vi "Eval X-Y(t).vi"(4 "Formulas":string[](array[string])=["", ""], 5 "end":dbl=1.0 format="%.2f", 6 "start":dbl format="%.2f", 7 "number of points":u32=10) -> (0 "error":i32, 1 "ticks":u32, 2 "Y":dbl[](array[numeric]) format="%.2f", 3 "X":dbl[](array[numeric]) format="%.2f")   [LabVIEW 2020, in "NI_Gmath.lvlib"]
doc: "Calculates the values of a function (f(t), g(t)), where t runs over an interval. Both components are given by <B>Formulas</B>. The t-values are chosen equidistantly in the interval."
uses:
  <vilib>/gmath/NI_Gmath.lvlib
panel:
  # "Example:\n\n number of points: 100 \n start: 0.0\n end: 1.0\n Formulas: sin(t*t)+t and exp(-t)"
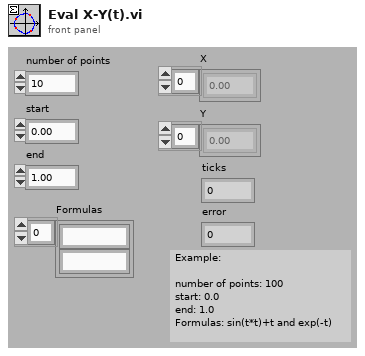
[diagram p1: front panel]
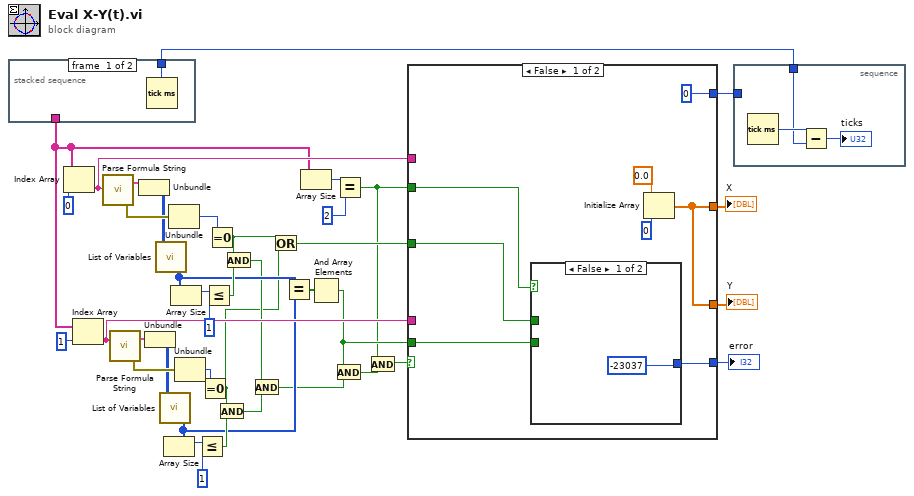
[diagram p0: block diagram]
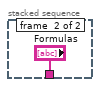
[diagram p2: hidden frame]
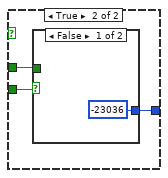
[diagram p3: hidden frame]
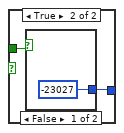
[diagram p4: hidden frame]
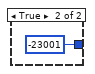
[diagram p5: hidden frame]
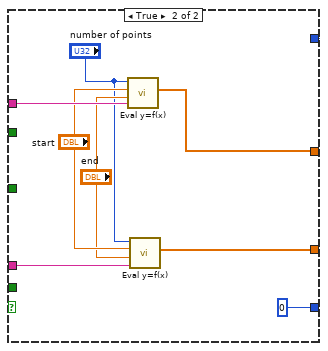
[diagram p6: hidden frame]
diagram:
  n1 = stacked-sequence {
    tunnel: [w40 _] -> w36
    tunnel: [_ "Formulas"] -> w1
    frame #0 {
      n2 = Tick Count (ms)() -> (millisecond timer value=w40:u32)
    }
    frame #1 {
    }
  }
  n3 = Index Array(array=w1, index=0) -> (element=w23:string)
  n4 = Index Array(array=w1, index=1) -> (element=w22:string)
  n5 = call <vilib>:"Parse Formula String.vi"("formula"=w23) -> ("error out"=w33:errorcluster, "Parsed Formula"=w5:cluster{"Table":i32[][], "Y Values":dbl[]})  [unwired: 1 in]
  n6 = call <vilib>:"Parse Formula String.vi"("formula"=w22) -> ("error out"=w26:errorcluster, "Parsed Formula"=w3:cluster{"Table":i32[][], "Y Values":dbl[]})  [unwired: 1 in]
  n7 = Unbundle(w5) -> ("Table"=w4:i32[][])  [unwired: 1 out]
  n8 = Unbundle(w3) -> ("Table"=w2:i32[][])  [unwired: 1 out]
  n9 = call <vilib>:"List of Variables.vi"("Table"=w4) -> ("List of variables"=w20:i32[])
  n10 = call <vilib>:"List of Variables.vi"("Table"=w2) -> ("List of variables"=w19:i32[])
  n11 = Array Size(array=w19) -> (size(s)=w24:i32)
  n12 = Unbundle(w33) -> ("code"=w32:i32)  [unwired: 2 out]
  n13 = Array Size(array=w20) -> (size(s)=w35:i32)
  n14 = Unbundle(w26) -> ("code"=w27:i32)  [unwired: 2 out]
  n15 = Less Or Equal?(x=w24, y=1) -> (x <= y?=w28:bool)
  n16 = Equal To 0?(x=w27) -> (x = 0?=w12:bool)
  n17 = Less Or Equal?(x=w35, y=1) -> (x <= y?=w31:bool)
  n18 = Equal To 0?(x=w32) -> (x = 0?=w13:bool)
  n19 = And(x=w12, y=w28) -> (x .and. y?=w21:bool)
  n20 = And(x=w13, y=w31) -> (x .and. y?=w14:bool)
  n21 = And(x=w14, y=w21) -> (x .and. y?=w18:bool)
  n22 = Or(x=w13, y=w12) -> (x .or. y?=w11:bool)
  n23 = Equal?(x=w20, y=w19) -> (x = y?=w17:bool[])
  n24 = Array Size(array=w1) -> (size(s)=w10:i32)
  n25 = And Array Elements(Boolean array=w17) -> (logical AND=w15:bool)
  n26 = And(x=w15, y=w18) -> (x .and. y?=w8:bool)
  n27 = Equal?(x=w10, y=2) -> (x = y?=w6:bool)
  n28 = And(x=w6, y=w8) -> (x .and. y?=w7:bool)
  n29 = case shown="False" w7 {
    tunnel: [w46 w61] -> w39
    tunnel: [w46 w60] -> w38
    tunnel: [0 0] -> w37
    tunnel: w23 -> [_ w66]
    tunnel: w22 -> [_ w63]
    tunnel: [w44 0] -> w16
    tunnel: w15 -> [w45 _]
    tunnel: w11 -> [w43 _]
    tunnel: w6 -> [w42 _]
    frame False {
      n30 = case shown="False" w42 {
        tunnel: w43 -> [_ w53]
        tunnel: [-23037 w52] -> w44
        tunnel: w45 -> [_ w51]
        frame False {
        }
        frame True {
          n31 = case shown="False" w51 {
            tunnel: [-23036 w55] -> w52
            tunnel: w53 -> [_ w56]
            frame False {
            }
            frame True {
              n32 = case shown="False" w56 {
                tunnel: [-23027 -23001] -> w55
                frame False {
                }
                frame True {
                }
              }
            }
          }
        }
      }
      n33 = Initialize Array(0.0, 0) -> (w46:dbl[])
    }
    frame True {
      n34 = call <vilib>:"Eval y=f(x).vi"("formula"=w66, "end"="end", "start"="start", "number of points"="number of points") -> ("Y Values"=w61:dbl[])  [unwired: 3 out]
      n35 = call <vilib>:"Eval y=f(x).vi"("formula"=w63, "end"="end", "start"="start", "number of points"="number of points") -> ("Y Values"=w60:dbl[])  [unwired: 3 out]
    }
  }
  "X" <- w39
  "Y" <- w38
  "error" <- w16
  n36 = stacked-sequence {
    tunnel: w37 -> [_]
    tunnel: w36 -> [w68]
    frame #0 {
      n37 = Tick Count (ms)() -> (millisecond timer value=w69:u32)
      n38 = Subtract(x=w69, y=w68) -> (x-y=→"ticks":u32)
    }
  }
